vi "DP-Acquire One.vi"(0 "State":T2, 2 "queue":refnum<queue>, 7 "level series":T1, 9 "iLevel":i32, 11 "error in (no error)":errorcluster, 12 "L2":dbl format="%#_13g") -> (4 "Error?":bool, 8 "Magnitude":dbl[](array[numeric]), 10 "Phase":dbl[](array[numeric]), 13 "waveform":cluster{i32, "dx":dbl, "Array":dbl[]}, 14 "aborted":bool, 15 "error out":errorcluster)   [LabVIEW 2020]
uses:
  Typedefs/DP-Runtime State.ctl
  Typedefs/DP-Queue Data.ctl
  Typedefs/DP-Parameters.ctl
  Typedefs/DP-Stimulus Params.ctl
  Typedefs/DP-Response Params.ctl
  Typedefs/DP-Level Series Info.ctl
  epl-vi-lib/PXI DAQ VIs/AIDI/Typedefs/AIDI-Action.ctl
  epl-vi-lib/PXI DAQ VIs/AODO/Typedefs/AODO-Action.ctl
  afcfbcde-8fef-4170-88b9-8379dbc42e1a.vi
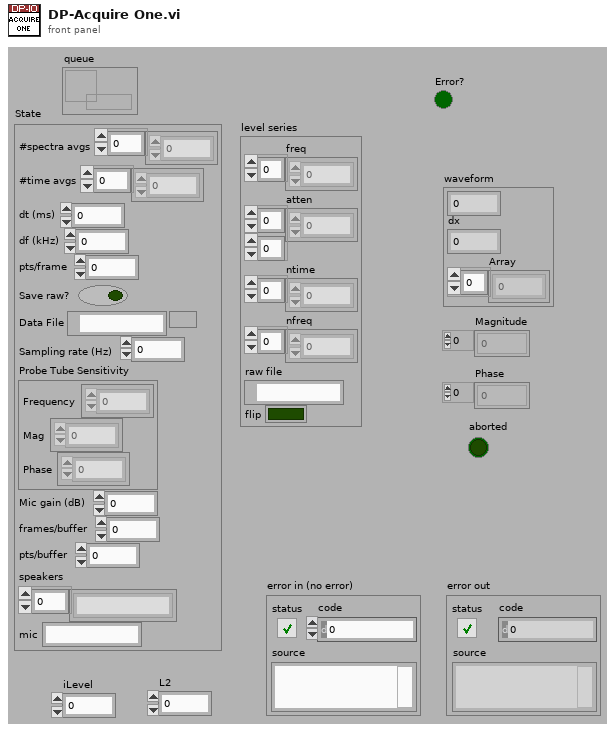
[diagram p1: front panel]
types:
  T1 = typedef "DP-Level Series Info.ctl" = cluster{"freq":dbl[], "atten":dbl[][], "ntime":i32[], "nfreq":i32[], "raw file":path, "flip":bool}
  T2 = typedef "DP-Runtime State.ctl" = cluster{"#spectra avgs":i32[], "#time avgs":i32[], "dt (ms)":dbl, "df (kHz)":dbl, "pts/frame":i32, "Save raw?":bool, "Data File":path, "Sampling rate (Hz)":dbl, "Probe Tube Sensitivity":cluster{"Frequency":dbl[], "Mag":dbl[], "Phase":dbl[]}, "Mic gain (dB)":dbl, "frames/buffer":i32, "pts/buffer":i32, "speakers":string[], "mic":string}
  T3 = typedef "AODO-Action.ctl" = enum16{"Configure", "Initialize", "Start", "Write", "Clean up", "Init & Start", "Config & Test", "Position", "Set AO Gains", "Zero", "Prime", "Status"}
  T4 = typedef "AIDI-Action.ctl" = enum16{"Configure", "Initialize", "Start", "Read", "Clean up", "Init & Start", "Config & Test", "Position", "Skip"}
  T5 = cluster{i32, "sine wave":dbl[][], "Array out":dbl[][]}
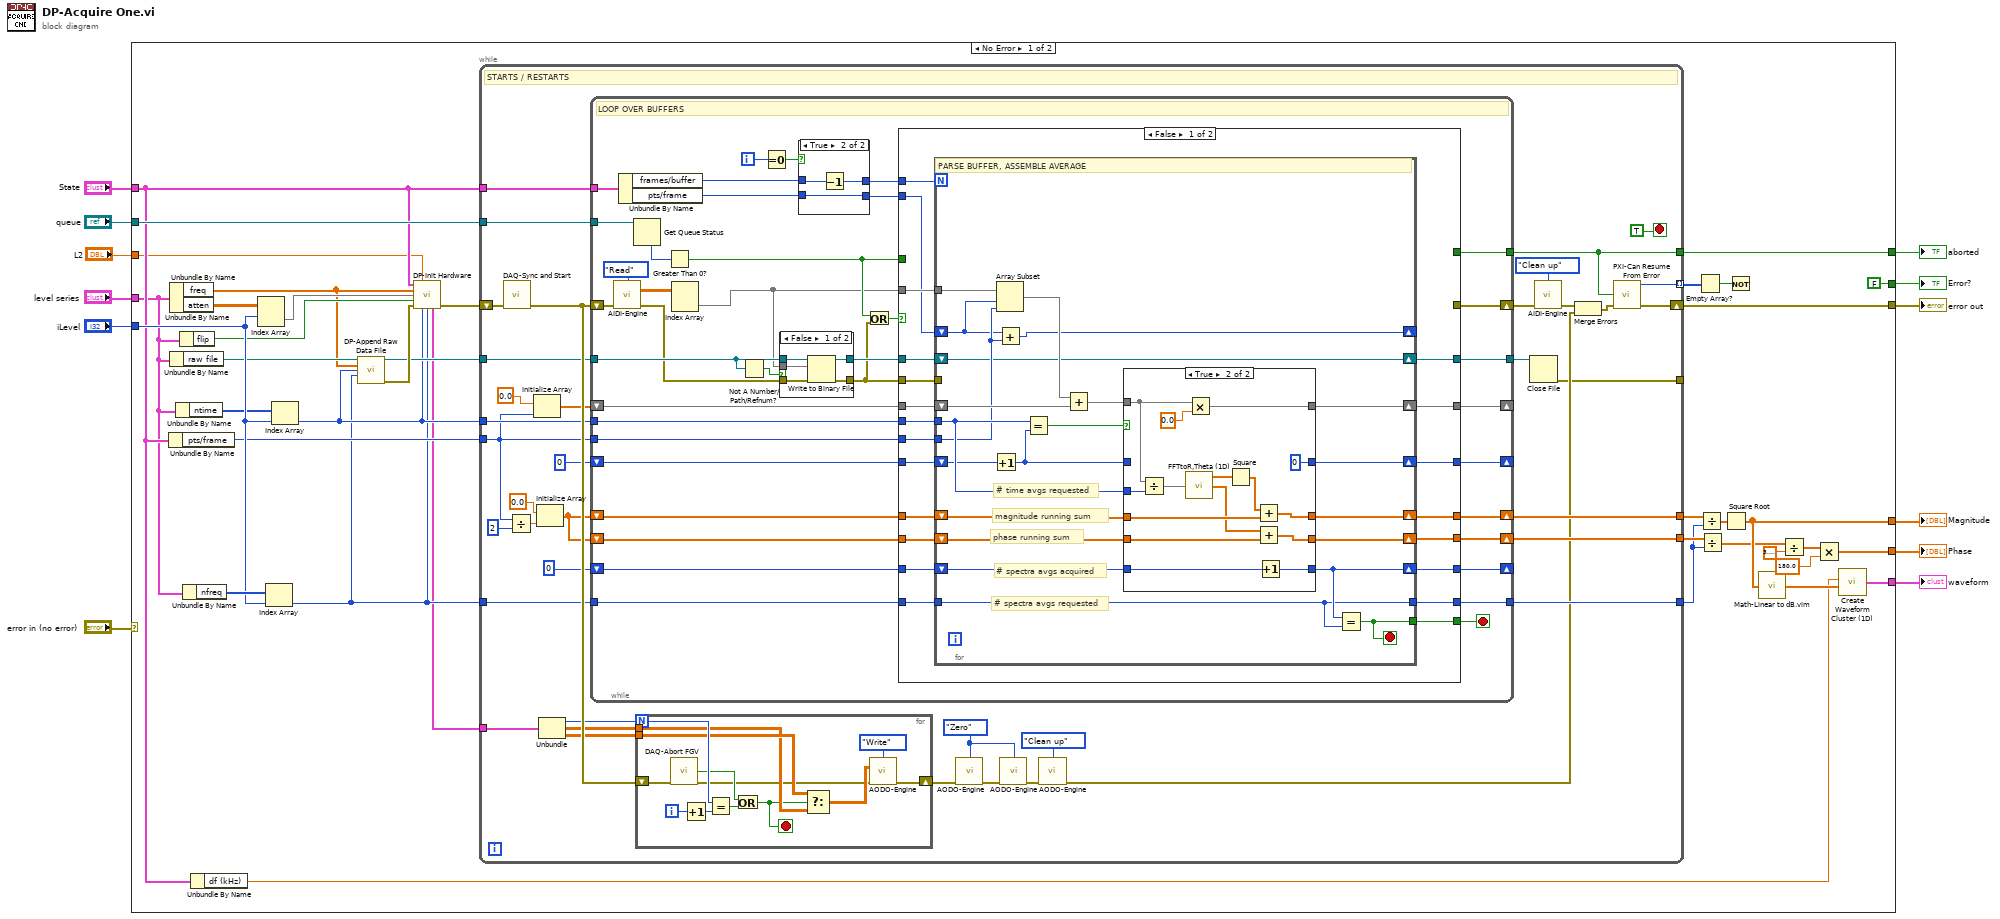
[diagram p0: block diagram]
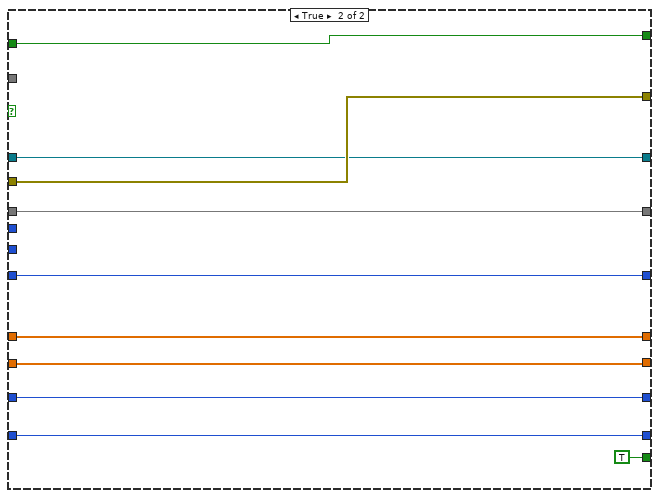
[diagram p3: hidden frame]
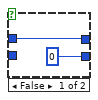
[diagram p4: hidden frame]
diagram:
  n1 = case shown="No Error" "error in (no error)" {
    selector: "error in (no error)" -> [_ w225]
    tunnel: [w49 _] -> w12
    tunnel: [w48 _] -> w11
    tunnel: "queue" -> [w47 _]
    tunnel: [w46 _] -> w10
    tunnel: "State" -> [w25 _]
    tunnel: [w45 w225] -> w3
    tunnel: [FALSE _] -> w8
    tunnel: "iLevel" -> [w37 _]
    tunnel: "level series" -> [w22 _]
    tunnel: [w27 _] -> w2
    tunnel: "L2" -> [w13 _]
    frame No Error {
      n2 = Unbundle By Name(w25) -> ("pts/frame"=w28:i32)
      n3 = Unbundle By Name(w22) -> ("freq"=w29:dbl[], "atten"=w35:dbl[][])
      n4 = Unbundle By Name(w22) -> ("raw file"=w32:path)
      n5 = Unbundle By Name(w22) -> ("ntime"=w23:i32[])
      n6 = Unbundle By Name(w22) -> ("flip"=w34:bool)
      n7 = Unbundle By Name(w22) -> ("nfreq"=w38:i32[])
      n8 = Unbundle By Name(w25) -> ("df (kHz)"=w26:dbl)
      n9 = Index Array(array=w35, index (row)=w37) -> (element=w33:dbl[])  [unwired: 1 in]
      n10 = Index Array(array=w38, index=w37) -> (element=w20:i32)
      n11 = Index Array(array=w23, index=w37) -> (element=w21:i32)
      n12 = call "DP-Append Raw Data File.vi"("raw file"=w32, "freq"=w29, "ntime"=w21, "nfreq"=w20) -> ("Byte Stream File out"=w30:refnum<file>, "error out"=w31:errorcluster)  [unwired: 10 in]
      n13 = call "DP-Init Hardware.vi"("State in"=w25, "L2"=w13, "freq"=w29, "atten"=w33, "flip"=w34, "error in (no error)"=w31, "ntime"=w21, "nfreq"=w20) -> ("stim"=w19:T5, "error out"=w36:errorcluster)  [unwired: 6 in]
      n14 = while {
        tunnel: [w87] -> w18
        tunnel: w28 -> [w72]
        tunnel: w47 -> [w81]
        tunnel: [w80] -> w17
        tunnel: w20 -> [w79]
        tunnel: [w78] -> w16
        tunnel: [w76] -> w15 mode=indexing
        tunnel: w21 -> [w75]
        tunnel: w30 -> [w73]
        shift-right: [w77] -> w45
        shift-left: w36 -> [w74]
        tunnel: w25 -> [w71]
        tunnel: [w52] -> w27
        tunnel: w19 -> [w56]
        tunnel: [w53] -> _
        stop <- TRUE stop-if-true
        w58 = AODO-Action."Zero" ("Action")
        # "STARTS / RESTARTS"
        n15 = call "DAQ-Sync and Start.vi"("error in (no error)"=w74) -> ("error out"=w88:errorcluster)  [unwired: 14 in]
        n16 = Divide(x=w72, y=2) -> (x/y=w82:dbl)
        n17 = Initialize Array(0.0, w72) -> (w85:dbl[])
        n18 = Initialize Array(0.0, w82) -> (w68:dbl[])
        n19 = Unbundle(w56) -> (w59:i32, "sine wave"=w60:dbl[][], "Array out"=w61:dbl[][])
        n20 = while {
          tunnel: w81 -> [w112]
          tunnel: w79 -> [w135]
          tunnel: [w134] -> w78
          tunnel: w75 -> [w133]
          tunnel: w73 -> [w130]
          shift-right: [w138] -> w66
          shift-left: w88 -> [w132]
          tunnel: w72 -> [w125]
          tunnel: w71 -> [w124]
          shift-right: [w122] -> _
          shift-left: 0 -> [w123]
          shift-right: [w120] -> _
          shift-left: 0 -> [w121]
          shift-right: [w119] -> _
          shift-left: w85 -> [w137]
          shift-right: [w139] -> w87
          shift-left: w68 -> [w107]
          shift-right: [w136] -> w80
          shift-left: w68 -> [w106]
          tunnel: [w104] -> w52
          tunnel: [w103] -> w54
          i -> [w118]
          stop <- w105 stop-if-true
          # "LOOP OVER BUFFERS"
          n21 = call "AIDI-Engine.vi"("Action"=AIDI-Action."Read", "error in (no error)"=w132) -> ("AI"=w127:dbl[][], "error out"=w128:errorcluster)  [unwired: 8 in, 4 out]
          n22 = Unbundle By Name(w124) -> ("frames/buffer"=w117:i32, "pts/frame"=w113:i32)
          n23 = Get Queue Status(queue=w112) -> (# elements in queue=w111:i32)  [unwired: 2 in, 7 out]
          n24 = Greater Than 0?(x=w111) -> (x > 0?=w108:bool)
          n25 = Index Array(array=w127) -> (element=w102:dbl[])  [unwired: 2 in]
          n26 = Not A Number/Path/Refnum?(number/path/refnum=w130) -> (NaN/Path/Refnum?=w129:bool)
          n27 = Equal To 0?(x=w118) -> (x = 0?=w116:bool)
          n28 = case shown="False" w129 {
            tunnel: w130 -> [w222 w223]
            tunnel: w128 -> [w221 w224]
            tunnel: w102 -> [w220 _]
            tunnel: [w219 w224] -> w110
            tunnel: [w218 w223] -> w126
            frame False {
              n29 = Write to Binary File(file (use dialog)=w222, data=w220, error in=w221) -> (refnum out=w218:refnum<file>, error out=w219:errorcluster)  [unwired: 3 in, 1 out]
            }
            frame True {
            }
          }
          n30 = case shown="True" w116 {
            tunnel: w117 -> [w214 w217]
            tunnel: [w214 w216] -> w115
            tunnel: [0 w215] -> w114
            tunnel: w113 -> [_ w215]
            frame False {
            }
            frame True {
              n31 = Decrement(x=w217) -> (x-1=w216:i32)
            }
          }
          n32 = Or(x=w108, y=w110) -> (x .or. y?=w109:bool)
          n33 = case shown="False" w109 {
            tunnel: [w160 w209] -> w139
            tunnel: [_ w212] -> w138
            tunnel: w137 -> [w159 w211]
            tunnel: w106 -> [w141 w208]
            tunnel: [w158 w208] -> w136
            tunnel: w135 -> [w157 w206]
            tunnel: [w156 w206] -> w134
            tunnel: w133 -> [w155 _]
            tunnel: w126 -> [w154 w203]
            tunnel: w102 -> [w153 _]
            tunnel: w125 -> [w152 _]
            tunnel: w123 -> [w151 w207]
            tunnel: [w150 w207] -> w122
            tunnel: w121 -> [w149 w210]
            tunnel: [w148 w210] -> w120
            tunnel: [w147 w211] -> w119
            tunnel: w115 -> [w146 _]
            tunnel: w114 -> [w145 _]
            tunnel: w110 -> [w144 w212]
            tunnel: w108 -> [_ w204]
            tunnel: w107 -> [w142 w209]
            tunnel: [w143 TRUE] -> w105
            tunnel: [_ w204] -> w104
            tunnel: [w140 w203] -> w103
            frame False {
              n34 = for {
                N: w146 -> [_]
                tunnel: w155 -> [w179]
                shift-right: [w181] -> w160
                shift-left: w142 -> [w182]
                tunnel: w144 -> [_]
                shift-right: [w178] -> w158
                shift-left: w141 -> [w177]
                shift-right: [w175] -> w150
                shift-left: w151 -> [w176]
                tunnel: w157 -> [w174]
                tunnel: [w174] -> w156
                tunnel: w153 -> [w173]
                tunnel: w152 -> [w172]
                shift-right: [w163] -> w148
                shift-left: w149 -> [w171]
                shift-right: [w168] -> _
                shift-left: w145 -> [w169]
                shift-right: [w165] -> w147
                shift-left: w159 -> [w180]
                tunnel: [w162] -> w143
                shift-right: [w161] -> w140
                shift-left: w154 -> [w161]
                stop <- w162 stop-if-true
                # "phase running sum"
                # "# spectra avgs acquired"
                # "# spectra avgs requested"
                # "# time avgs requested"
                # "magnitude running sum"
                # "PARSE BUFFER, ASSEMBLE AVERAGE"
                n35 = Increment(x=w171) -> (x+1=w164:i32)
                n36 = Array Subset(array=w173, index=w169, length=w172) -> (w170:dbl[])
                n37 = Add(x=w169, y=w172) -> (x+y=w168:i32)
                n38 = Equal?(x=w179, y=w164) -> (x = y?=w166:bool)
                n39 = Add(x=w170, y=w180) -> (x+y=w167:dbl[])
                n40 = case shown="True" w166 {
                  tunnel: w182 -> [w186 w202]
                  tunnel: [w186 w201] -> w181
                  tunnel: w179 -> [_ w200]
                  tunnel: [w185 w198] -> w178
                  tunnel: w177 -> [w185 w196]
                  tunnel: w176 -> [w184 w194]
                  tunnel: [w184 w193] -> w175
                  tunnel: w167 -> [w187 w191]
                  tunnel: [w187 w190] -> w165
                  tunnel: w164 -> [w183 _]
                  tunnel: [w183 0] -> w163
                  frame False {
                  }
                  frame True {
                    n41 = Divide(x=w191, y=w200) -> (x/y=w199:dbl[])
                    n42 = call "FFTtoR,Theta (1D).VI"("X"=w199) -> ("+Freq. Mag of FFT"=w195:dbl[], "+Freq Theta of FFT"=w197:dbl[])  [unwired: 1 in]
                    n43 = Multiply(x=w191, y=0.0) -> (x*y=w190:dbl[])
                    n44 = Square(x=w195) -> (x^2=w192:dbl[])
                    n45 = Add(x=w192, y=w202) -> (x+y=w201:dbl[])
                    n46 = Add(x=w197, y=w196) -> (x+y=w198:dbl[])
                    n47 = Increment(x=w194) -> (x+1=w193:i32)
                  }
                }
                n48 = Equal?(x=w175, y=w174) -> (x = y?=w162:bool)
              }
            }
            frame True {
            }
          }
        }
        n49 = for {
          N: w59 -> [w99]
          tunnel: w60 -> [w95]
          tunnel: w61 -> [w96]
          shift-right: [w90] -> w64
          shift-left: w88 -> [w89]
          i -> [w101]
          stop <- w94 stop-if-true
          n50 = call "DAQ-Abort FGV.vi"("error in (no error)"=w89) -> ("Stop"=w97:bool, "Errors"=w91:errorcluster)  [unwired: 12 in, 1 out]
          n51 = Increment(x=w101) -> (x+1=w100:i32)
          n52 = Equal?(x=w99, y=w100) -> (x = y?=w98:bool)
          n53 = Or(x=w97, y=w98) -> (x .or. y?=w94:bool)
          n54 = Select(t=w96, s=w94, f=w95) -> (s? t:f=w92:dbl[][])
          n55 = call "AODO-Engine.vi"("Action"=AODO-Action."Write", "AO"=w92, "error in (no error)"=w91) -> ("error out"=w90:errorcluster)  [unwired: 7 in, 5 out]
        }
        n56 = call "AODO-Engine.vi"("Action"=w58, "error in (no error)"=w64) -> ("error out"=w62:errorcluster)  [unwired: 8 in, 5 out]
        n57 = call "AODO-Engine.vi"("Action"=w58, "error in (no error)"=w62) -> ("error out"=w63:errorcluster)  [unwired: 8 in, 5 out]
        n58 = call "AODO-Engine.vi"("Action"=AODO-Action."Clean up", "error in (no error)"=w63) -> ("error out"=w55:errorcluster)  [unwired: 8 in, 5 out]
        n59 = Close File(refnum=w54) -> (error out=w53:errorcluster)  [unwired: 1 in, 1 out]
        n60 = call "AIDI-Engine.vi"("Action"=AIDI-Action."Clean up", "error in (no error)"=w66) -> ("error out"=w65:errorcluster)  [unwired: 8 in, 5 out]
        n61 = Merge Errors(w65, w55) -> (w51:errorcluster)
        n62 = call "PXI-Can Resume From Error.vi"("Abort"=w52, "error in (no error)"=w51) -> ("code"=w76:i32, "error out"=w77:errorcluster)  [unwired: 11 in, 1 out]
      }
      n63 = Empty Array?(array=w15) -> (empty?=w24:bool)
      n64 = Divide(x=w18, y=w16) -> (x/y=w44:dbl[])
      n65 = Divide(x=w17, y=w16) -> (x/y=w42:dbl[])
      n66 = Square Root(x=w44) -> (sqrt(x)=w49:dbl[])
      n67 = Not(x=w24) -> ()  [unwired: 1 out]
      n68 = call "Math-Linear to dB.vim"("linear"=w49) -> ("dB"=w43:dbl[])
      n69 = Divide(x=w42, y=3.141592653589793) -> (x/y=w41:dbl[])
      n70 = Multiply(x=w41, y=180.0) -> (x*y=w46:dbl[])
      n71 = call "Create Waveform Cluster (1D).vi"("dx"=w26, "Y"=w43) -> ("waveform cluster"=w48:cluster{dbl, "dx":dbl, "Y":dbl[]})  [unwired: 3 in]
    }
    frame Error {
    }
  }
  "waveform" <- w11
  "Magnitude" <- w12
  "Phase" <- w10
  "Error?" <- w8
  "aborted" <- w2
  "error out" <- w3
